vi "Boiler_Startup_Control.vi"() -> ()   [LabVIEW 2023]
doc: "This is the Main Vi that performs the boiler startup operation."
uses:
  Controls/Boiler_Status_Indicators.ctl
  Controls/Queue_Operation_Select.ctl
  Controls/Timer_Operation_Select.ctl
  Controls/Boiler_Data.ctl
  Controls/State_and_Data.ctl
  Controls/Notifier_Operation_Select.ctl
  <vilib>/Utility/file.llb/Write Delimited Spreadsheet (string).vi
panel:
  out "Boiler_Status_Indicators":T1 caption="Boiler Status Indicators"
  in  "Stop":bool
  in  "Forced_Draft_Fan":bool caption="Forced Draft Fan"
  in  "Run_Interlock":bool caption="Run Interlock"
  in  "Flame_Sensor_Value":dbl(slide) caption="Flame Sensor Value [%]" scale=0.0..100.0
  in  "Fuel_Control_Valve":dbl(knob) caption="Fuel  Control Valve Position [% Open]" scale=0.0..100.0 scale format="%.1f"
  in  "Shutdown":bool
  in  "Pilot":bool
  in  "Start_Sequence":bool caption="Start Sequence"
  in  "Boiler_Reset":bool caption="Boiler Reset"
  out "Error_Out":errorcluster
  in  "Error_In":errorcluster
  # "Boiler Controls"
  # "Boiler Simulation Controls"
  # "Closed"
  # "On"
  # "Open"
  # "Off"
  # "Boiler Start-Up steps\nStep1 : Close the interlock and hit the reset button.\nStep2 : Press the start sequence to initiate the pre-purge. \nStep3 : After the pre-purge, press the pilot button to turn on the natural gas and pilot.\nStep4 : Adjust the flame sensor to prepare the boiler.\nStep5 : Turn on the forced draft fan, then add fuel to the boiler by adjusting the fuel control valve.\nStep6 :The boiler is now started up"
  # "Seconds"
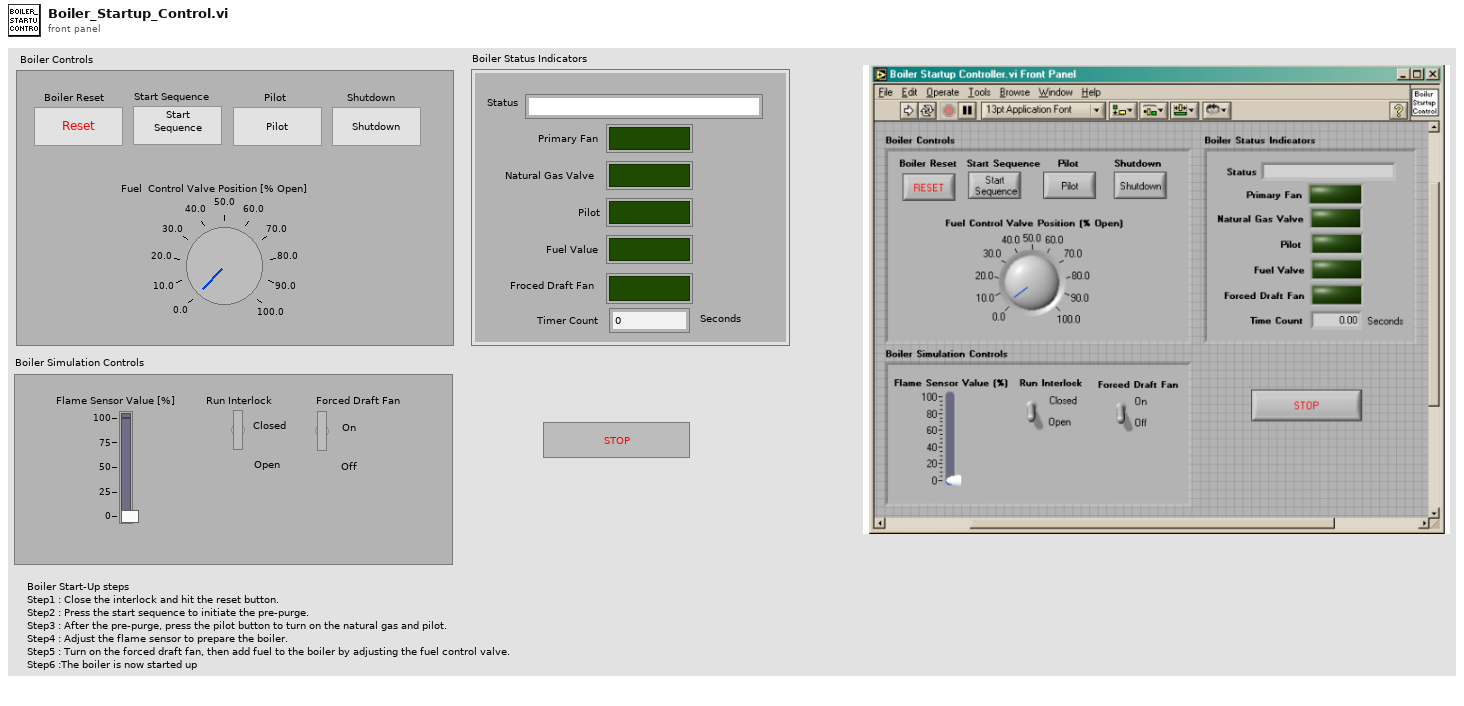
[diagram p1: front panel]
types:
  T1 = typedef "Boiler_Status_Indicators.ctl" = cluster{"Status":string, "Primary_Fan":bool, "Natural_Gas_Valve":bool, "Pilot":bool, "Fuel_Value":bool, "Froced_Draft_Fan":bool, "Timer_Count":dbl}
  T2 = typedef "Notifier_Operation_Select.ctl" = enum16{"Obtain_Notifier", "Send_Notification", "Get_Notification_Status", "Release_Notifier"}
  T3 = typedef "Queue_Operation_Select.ctl" = enum16{"Obtain_Queue", "Enqueue", "Enqueue_N", "Enqueue_at_First", "Dequeue", "Flush_Queue", "Release_Queue"}
  T4 = typedef "State_and_Data.ctl" = cluster{"State":string, "Event_Data":variant}
  T5 = typedef "Boiler_Data.ctl" = cluster{"Boiler_Status_Indicators":T1, "Start?":bool, "Pilot_On?":bool, "Blink_It?":bool, "Log_Timer_Time":bool, "ReInitialize":refnum<vi>[], "After_TimeOut_Call?":string, "Time_String":string, "Event_String":string, "Event_Data_String":string}
  T6 = typedef "Timer_Operation_Select.ctl" = enum16{"Start_Timer", "Pause_Timer", "Time_Out?", "Stop_Timer"}
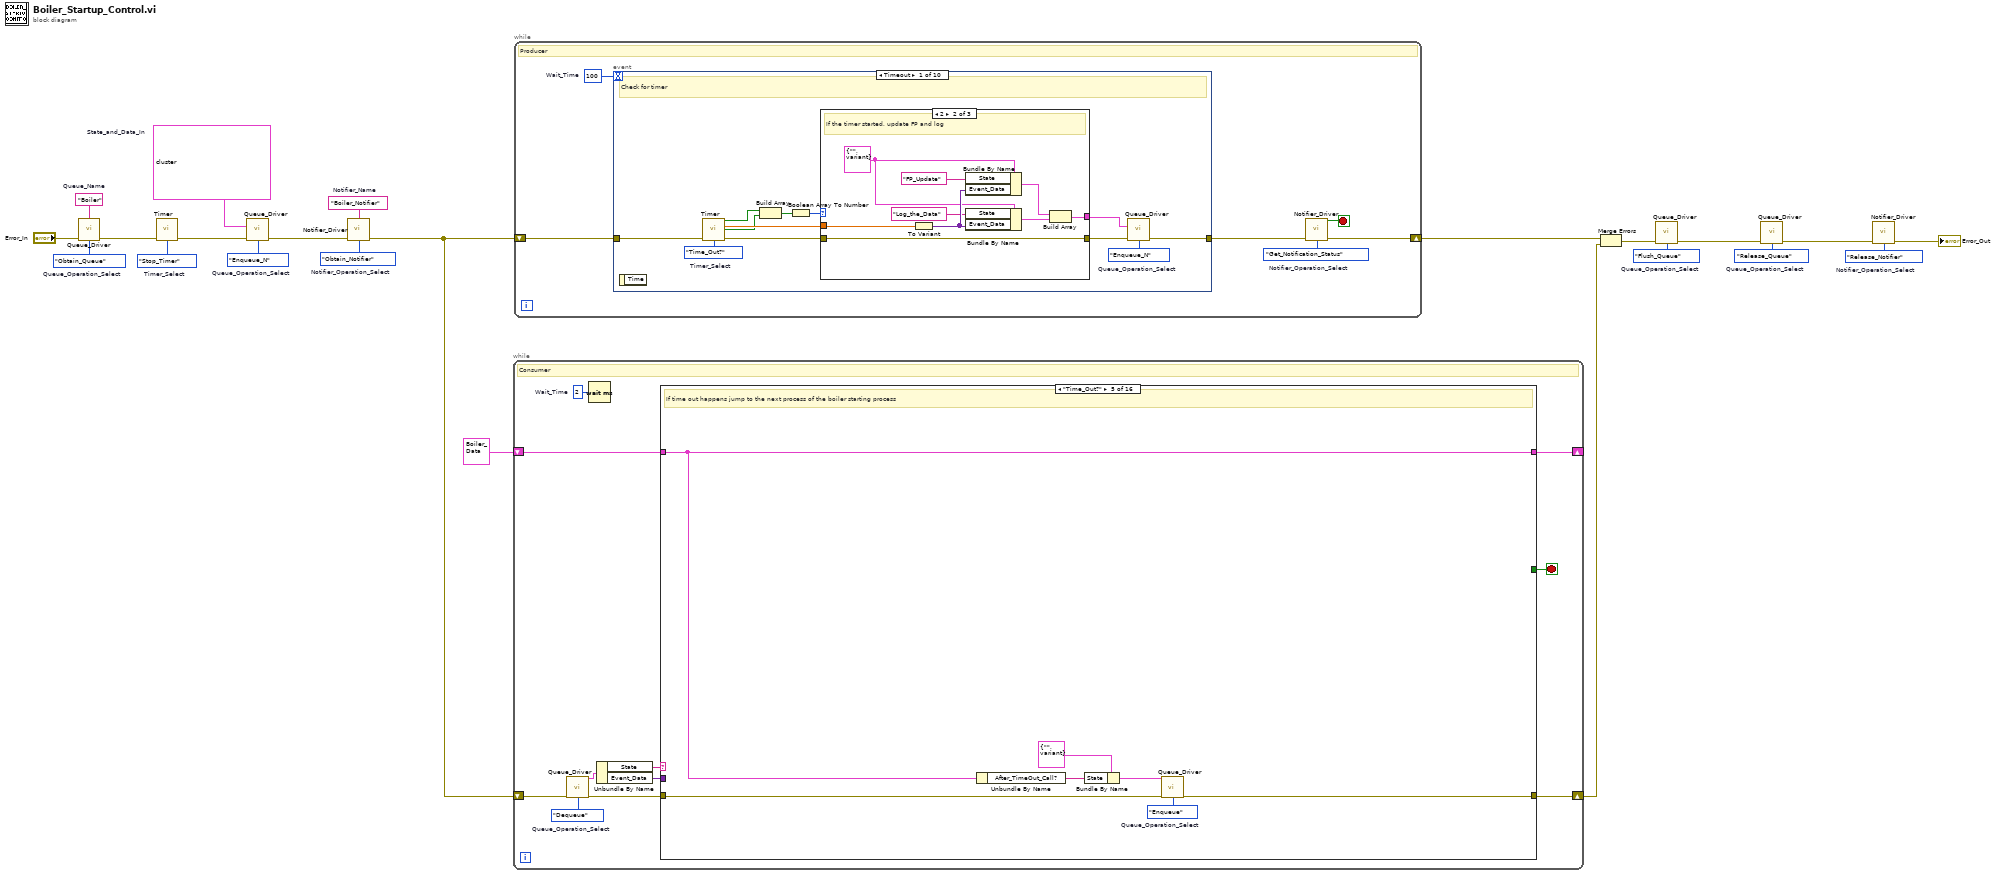
[diagram p0: block diagram]
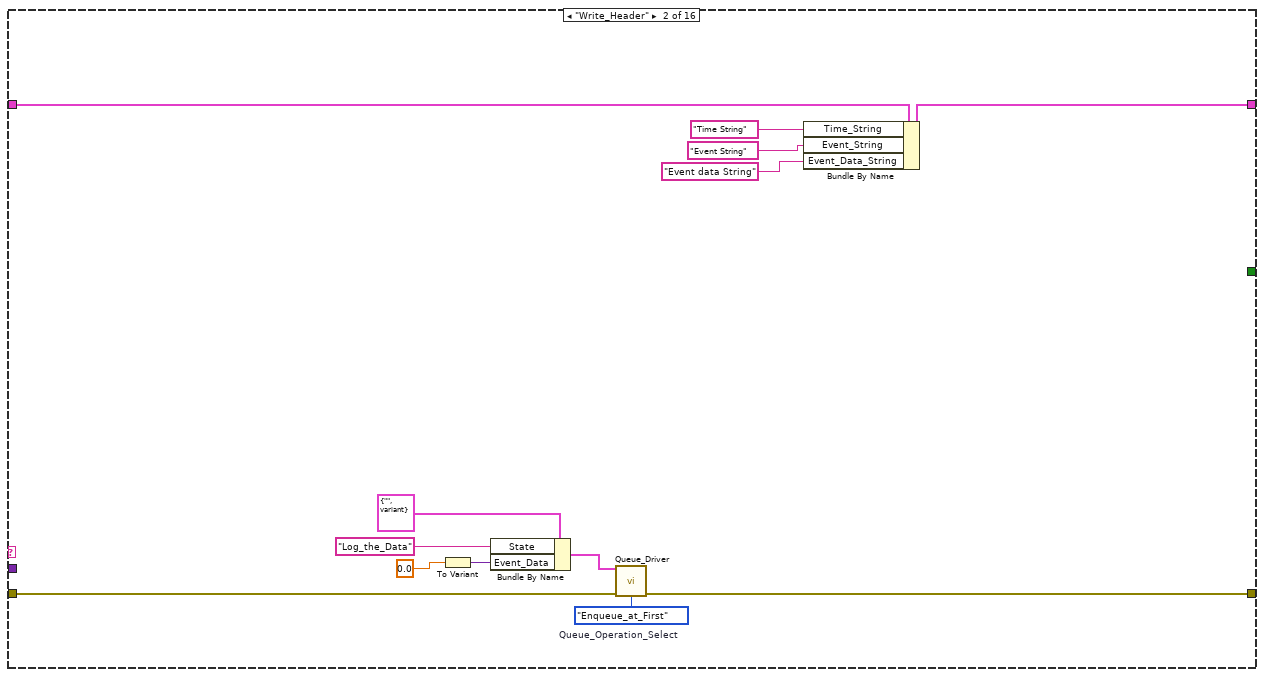
[diagram p3: hidden frame]
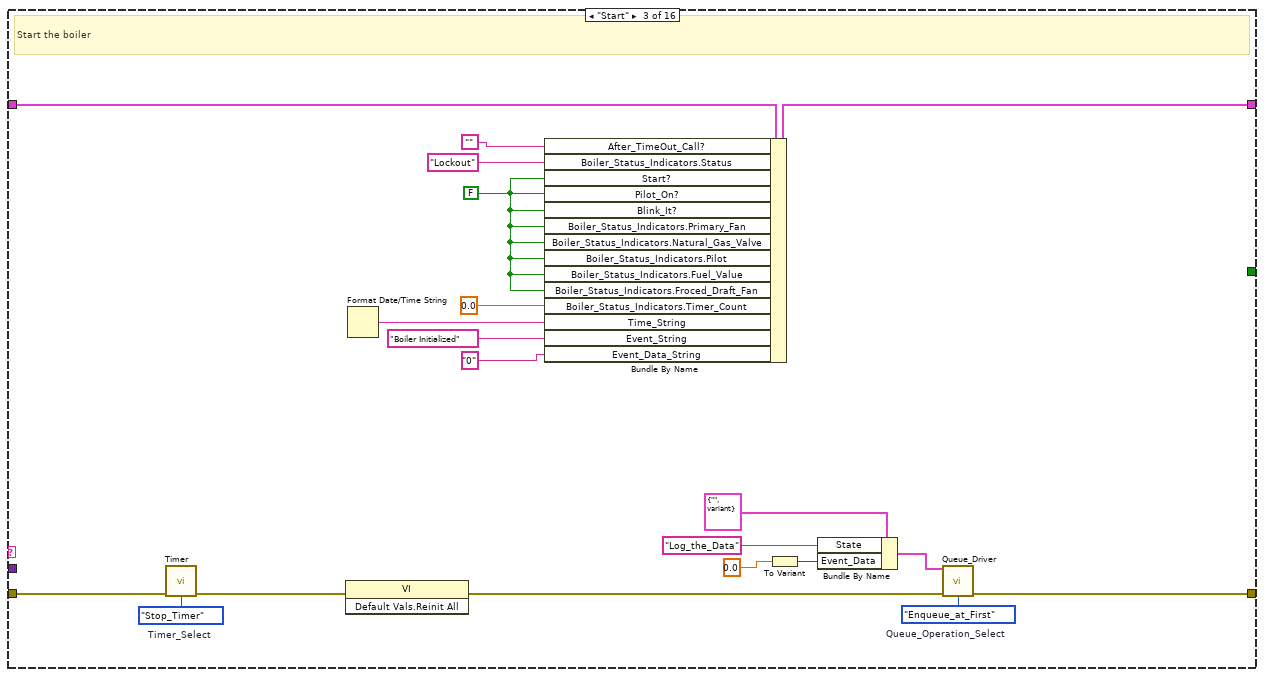
[diagram p4: hidden frame]
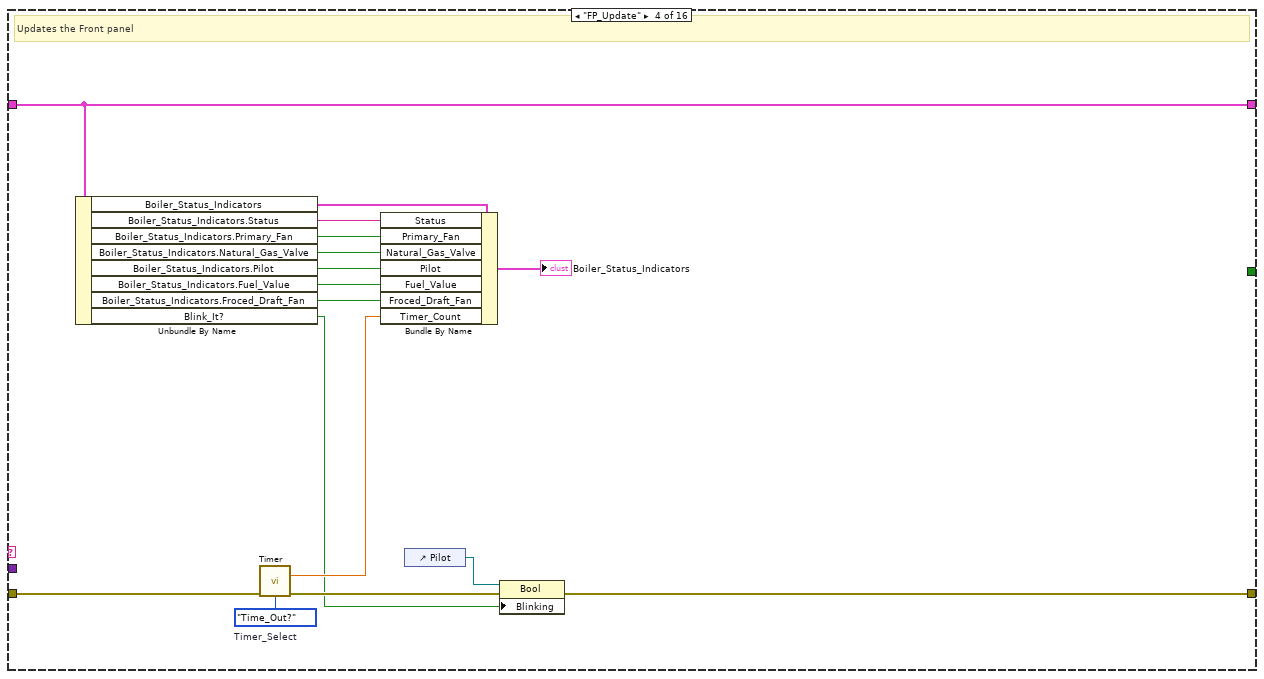
[diagram p5: hidden frame]
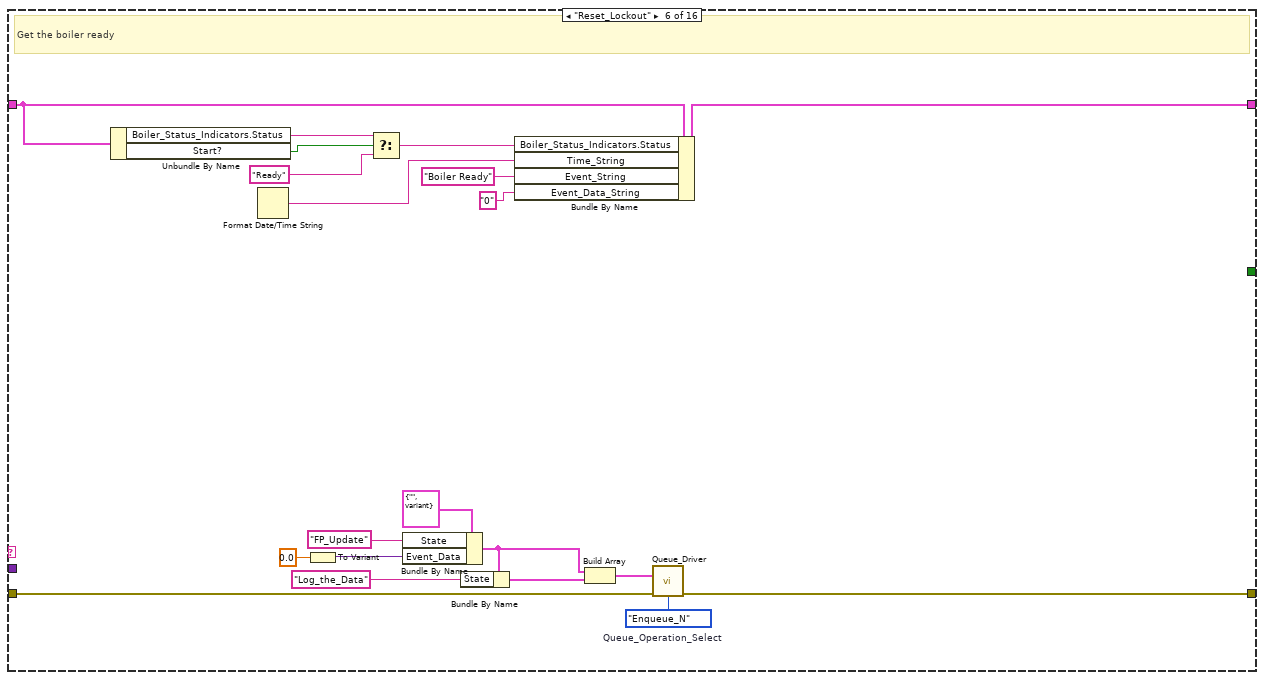
[diagram p6: hidden frame]
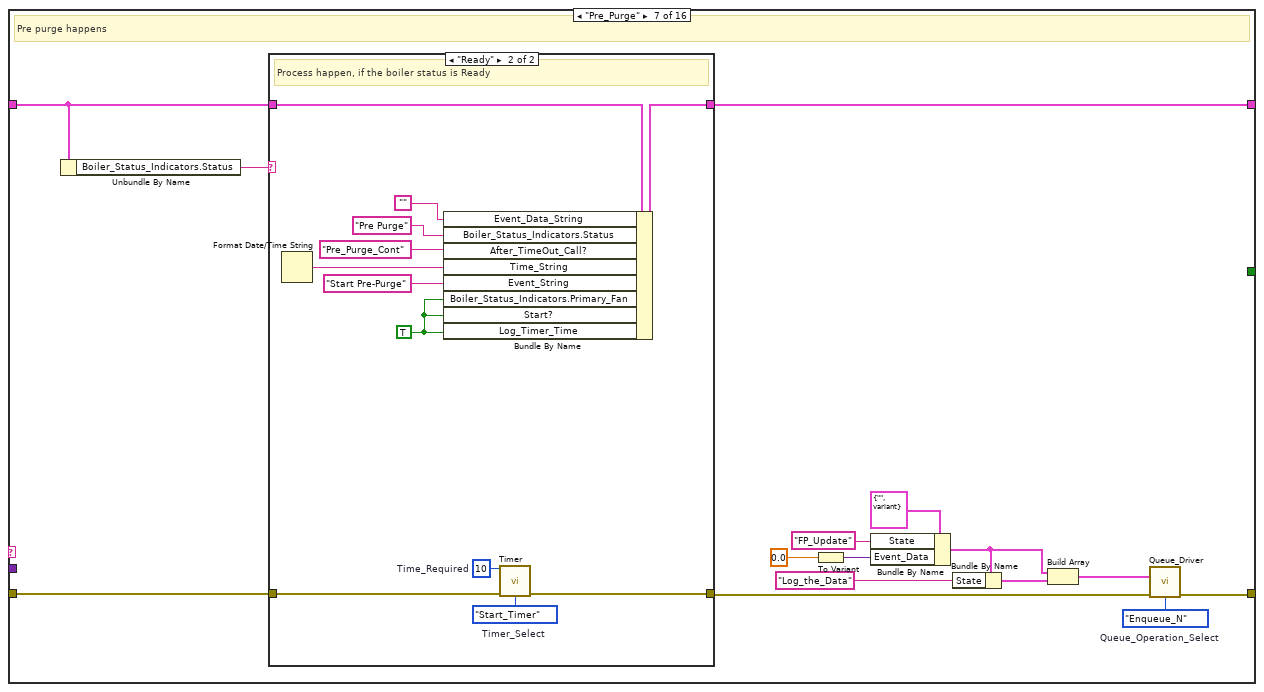
[diagram p7: hidden frame]
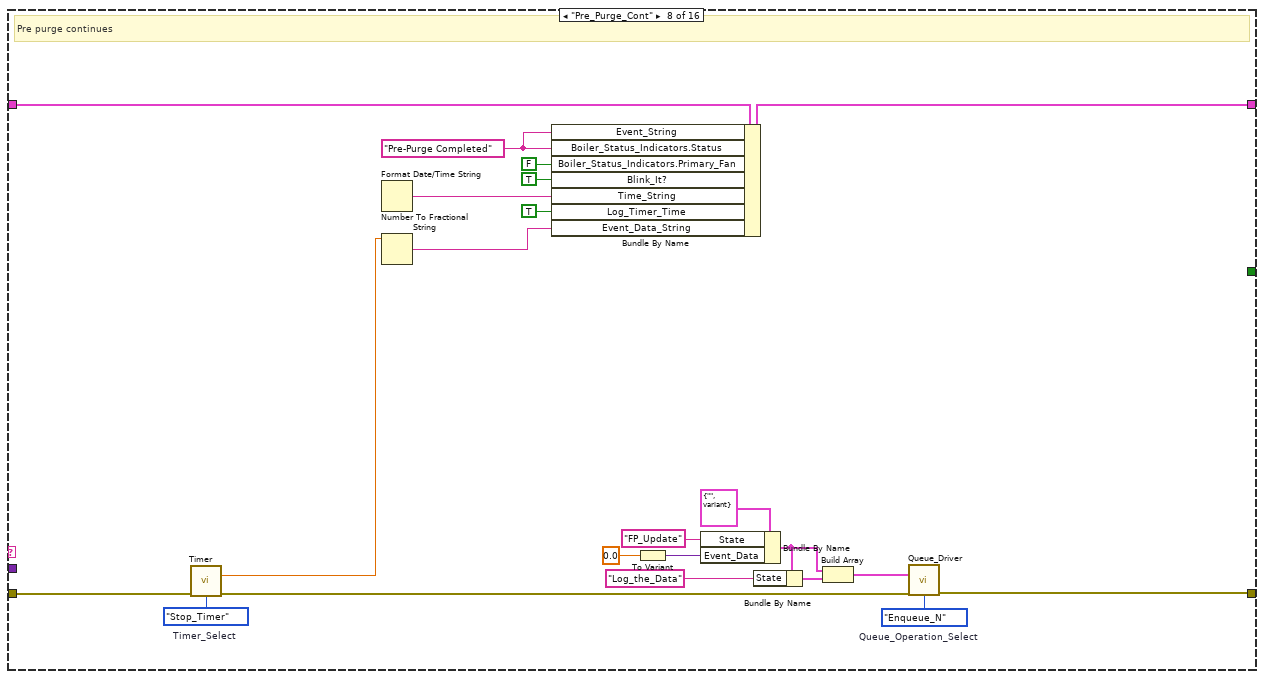
[diagram p9: hidden frame]
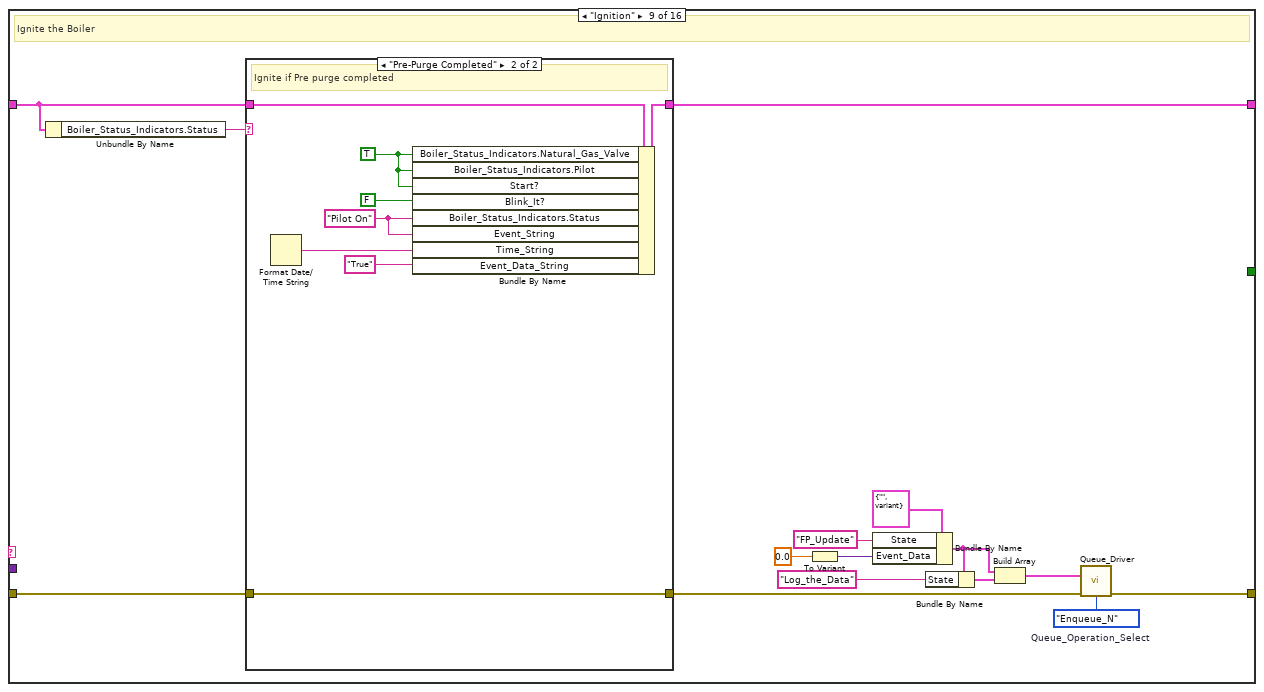
[diagram p10: hidden frame]
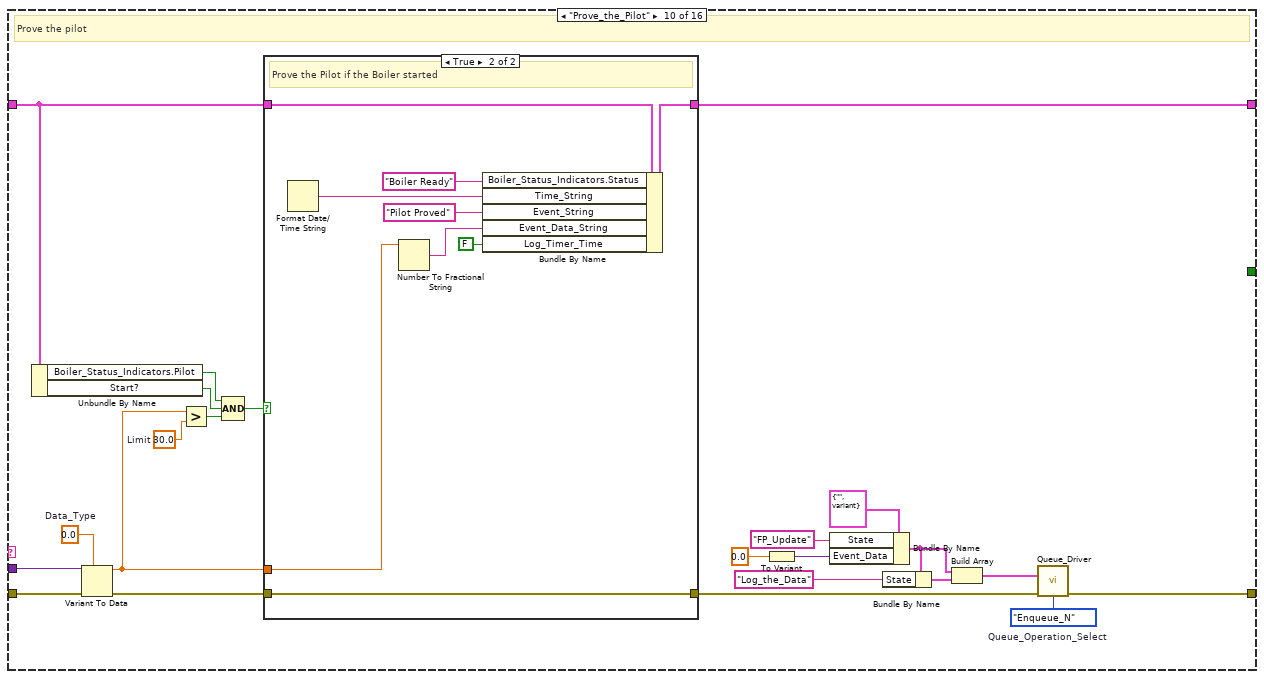
[diagram p12: hidden frame]
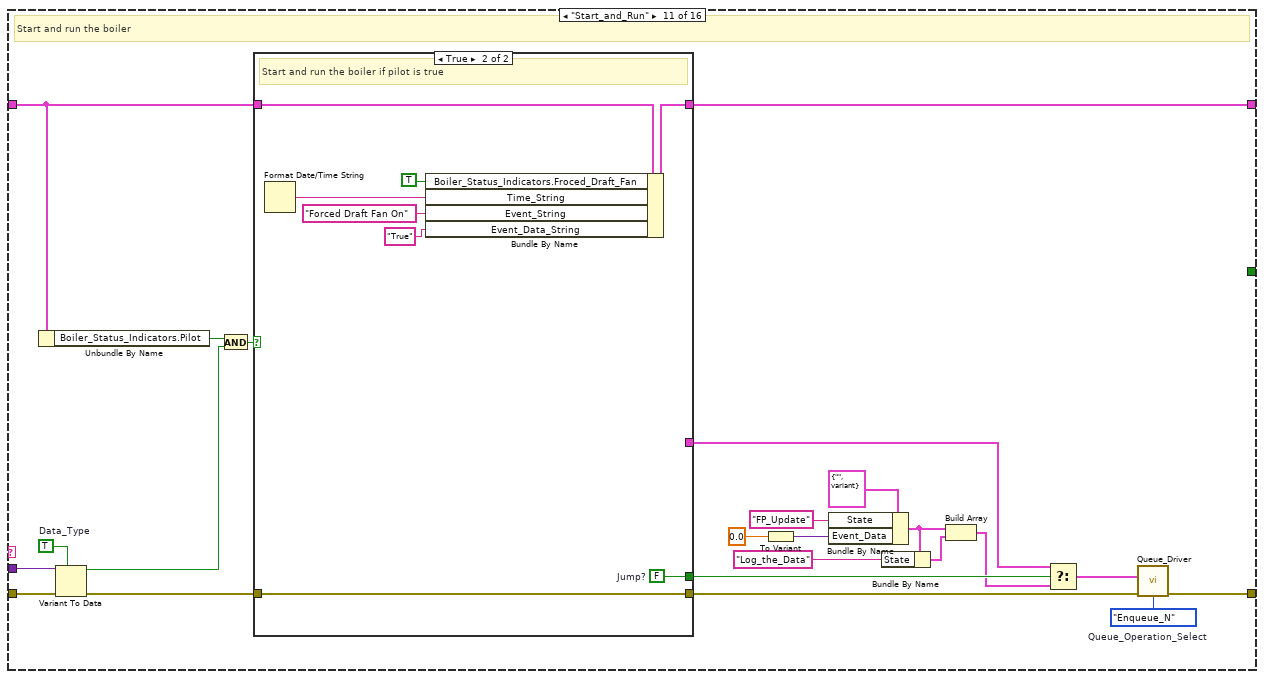
[diagram p14: hidden frame]
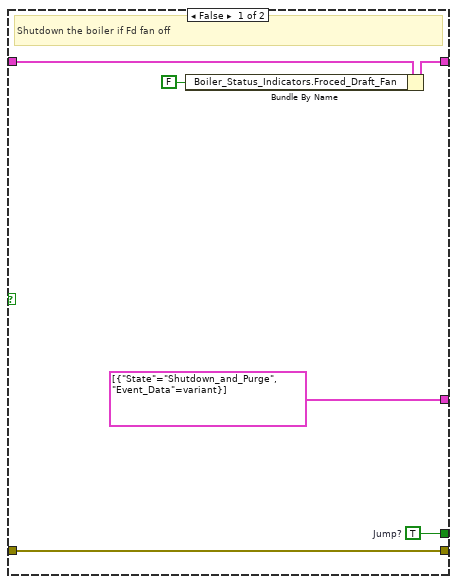
[diagram p15: hidden frame]
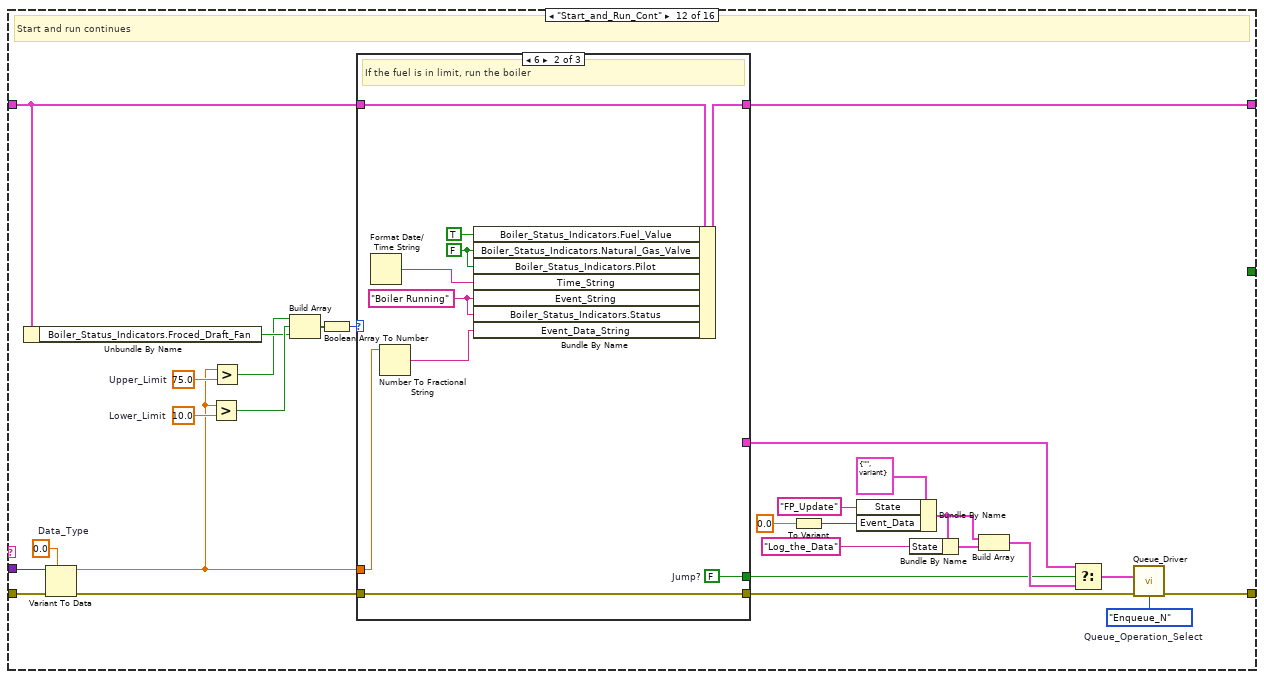
[diagram p16: hidden frame]
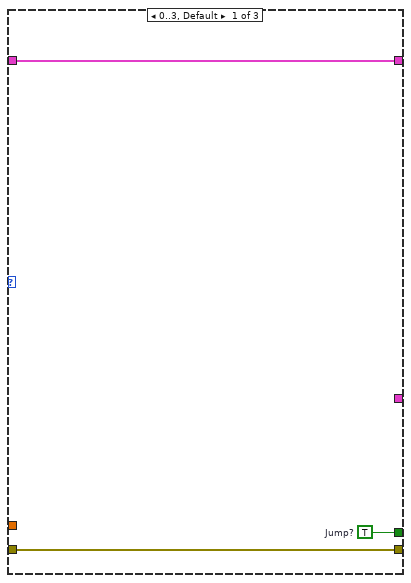
[diagram p17: hidden frame]
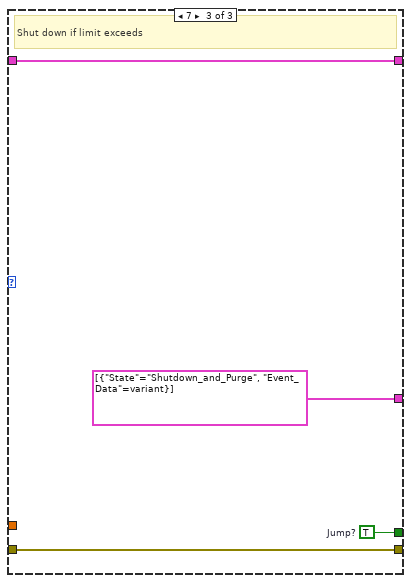
[diagram p18: hidden frame]
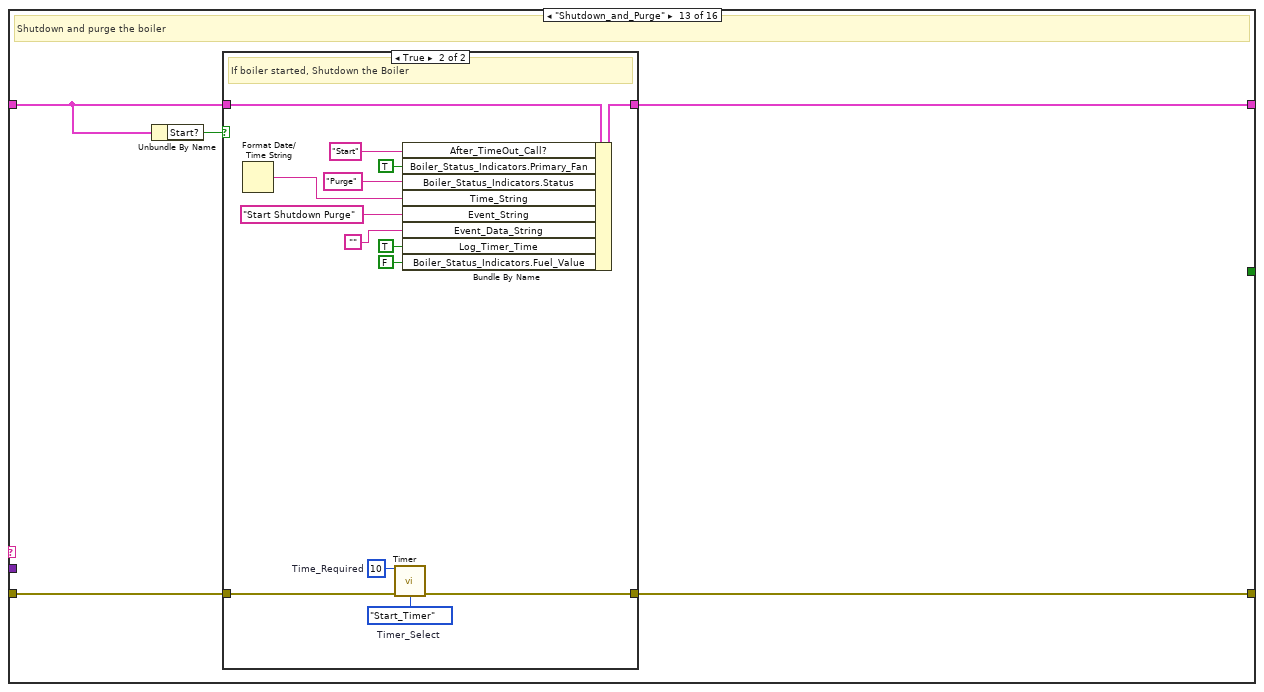
[diagram p19: hidden frame]
diagram:
  w5 = Notifier_Operation_Select."Release_Notifier"  # Notifier_Operation_Select
  w6 = Queue_Operation_Select."Release_Queue"  # Queue_Operation_Select
  w8 = Queue_Operation_Select."Flush_Queue"  # Queue_Operation_Select
  w10 = "Boiler_Notifier"  # Notifier_Name
  w11 = Notifier_Operation_Select."Obtain_Notifier"  # Notifier_Operation_Select
  w13 = T4[] [{"State"="Write_Header", "Event_Data"=variant}, {"State"="Start", "Event_Data"=variant}, {"State"="FP_Update", "Event_Data"=variant}]  # State_and_Data_In
  w14 = Queue_Operation_Select."Enqueue_N"  # Queue_Operation_Select
  w18 = Timer_Operation_Select."Stop_Timer"  # Timer_Select
  w19 = "Boiler"  # Queue_Name
  w20 = Queue_Operation_Select."Obtain_Queue"  # Queue_Operation_Select
  n1 = call "Queue_Driver.vi"("Queue_Name"=w19, "Error_In"="Error_In", "Queue_Operation_Select"=w20) -> ("Error_Out"=w21:errorcluster)  [unwired: 11 in, 1 out]
  n2 = call "Timer.vi"("Error_In"=w21, "Timer_Select"=w18) -> ("Error_Out"=w17:errorcluster)  [unwired: 10 in, 3 out]
  n3 = call "Queue_Driver.vi"("State_and_Data_In_N"=w13, "Error_In"=w17, "Queue_Operation_Select"=w14) -> ("Error_Out"=w15:errorcluster)  [unwired: 11 in, 1 out]
  n4 = call "Notifier_Driver.vi"("Notifier_Name"=w10, "Error_In"=w15, "Notifier_Operation_Select"=w11) -> ("Error_Out"=w12:errorcluster)  [unwired: 11 in, 1 out]
  n5 = while {
    shift-right: [w28] -> _
    shift-left: T5 {"Boiler_Status_Indicators"={"Status"="", "Primary_Fan"=FALSE, "Natural_Gas_Valve"=FALSE, "Pilot"=FALSE, "Fuel_Value"=FALSE, "Froced_Draft_Fan"=FALSE, "Timer_Count"=0.0}, "Start?"=TRUE, "Pilot_On?"=TRUE, "Blink_It?"=TRUE, "Log_Timer_Time"=FALSE, "ReInitialize"=[], "After_TimeOut_Call?"="", "Time_String"="", "Event_String"="", "Event_Data_String"=""} -> [w27]
    shift-right: [w23] -> w4
    shift-left: w12 -> [w33]
    stop <- w25 stop-if-true
    w24 = u32 2  # Wait_Time
    w31 = Queue_Operation_Select."Dequeue"  # Queue_Operation_Select
    # "Consumer"
    n6 = call "Queue_Driver.vi"("Error_In"=w33, "Queue_Operation_Select"=w31) -> ("State_and_Data_Out"=w30:T4, "Error_Out"=w32:errorcluster)  [unwired: 12 in]
    n7 = Wait (ms)(milliseconds to wait=w24) -> ()  [unwired: 1 out]
    n8 = Unbundle By Name(w30) -> ("State"=w29:string, "Event_Data"=w26:variant)
    n9 = case shown="\"Time_Out?\"" w29 {
      tunnel: w32 -> [w35 w48 w61 w84 w88 w95 w125 w159 w176 w210 w244 w284 w308 w343 w355 w364]
      tunnel: [w35 w42 w49 w69 w87 w94 w114 w141 w163 w189 w226 w262 w306 w347 w353 w359] -> w23
      tunnel: [w34 w46 w68 w83 w90 w111 w126 w162 w177 w201 w243 w286 w307 w344 w354 w375] -> w28
      tunnel: w27 -> [w34 w47 w67 w83 w90 w109 w124 w160 w175 w202 w242 w285 w305 w344 w354 w375]
      tunnel: w26 -> [_ _ _ _ _ _ _ _ _ w209 w239 w282 _ w342 _ _]
      tunnel: [_ _ _ _ _ _ _ _ _ _ _ _ _ _ w348 _] -> w25
      frame Default {
        # "Default"
      }
      frame "Write_Header" {
        w41 = Queue_Operation_Select."Enqueue_at_First"  # Queue_Operation_Select
        n10 = To Variant(anything=0.0) -> (Variant=w36:variant)
        n11 = Bundle By Name(cluster=T4 {"State"="", "Event_Data"=variant} ("State_and_Data_In"), "State"="Log_the_Data", "Event_Data"=w36) -> (w39:T4)
        n12 = call "Queue_Driver.vi"("State_and_Data_In"=w39, "Error_In"=w48, "Queue_Operation_Select"=w41) -> ("Error_Out"=w42:errorcluster)  [unwired: 11 in, 1 out]
        n13 = Bundle By Name(cluster=w47, "Time_String"="Time String", "Event_String"="Event String", "Event_Data_String"="Event data String") -> (w46:T5)
      }
      frame "Start" {
        w56 = Queue_Operation_Select."Enqueue_at_First"  # Queue_Operation_Select
        w58 = Timer_Operation_Select."Stop_Timer"  # Timer_Select
        w62 = FALSE ("Boiler_Status_Indicators.Primary_Fan")
        # "Start the boiler"
        n14 = call "Timer.vi"("Error_In"=w61, "Timer_Select"=w58) -> ("Error_Out"=w59:errorcluster)  [unwired: 10 in, 3 out]
        n15 = invoke on="Invoke Node" class="VI" method="Default Vals.Reinit All"(error in=w59) -> (error out=w50:errorcluster)  [unwired: 2 in, 2 out]
        n16 = Format Date/Time String() -> (date/time string=w57:string)  [unwired: 3 in]
        n17 = Bundle By Name(cluster=w67, "After_TimeOut_Call?"="" ("Empty String Constant"), "Boiler_Status_Indicators.Status"="Lockout", "Start?"=w62, "Pilot_On?"=w62, "Blink_It?"=w62, "Boiler_Status_Indicators.Primary_Fan"=w62, "Boiler_Status_Indicators.Natural_Gas_Valve"=w62, "Boiler_Status_Indicators.Pilot"=w62, "Boiler_Status_Indicators.Fuel_Value"=w62, "Boiler_Status_Indicators.Froced_Draft_Fan"=w62, "Boiler_Status_Indicators.Timer_Count"=0.0, "Time_String"=w57, "Event_String"="Boiler Initialized", "Event_Data_String"="0") -> (w68:T5)
        n18 = To Variant(anything=0.0) -> (Variant=w51:variant)
        n19 = Bundle By Name(cluster=T4 {"State"="", "Event_Data"=variant} ("State_and_Data_In"), "State"="Log_the_Data", "Event_Data"=w51) -> (w54:T4)
        n20 = call "Queue_Driver.vi"("State_and_Data_In"=w54, "Error_In"=w50, "Queue_Operation_Select"=w56) -> ("Error_Out"=w49:errorcluster)  [unwired: 11 in, 1 out]
      }
      frame "FP_Update" {
        w74 = Timer_Operation_Select."Time_Out?"  # Timer_Select
        # "Updates the Front panel"
        n21 = Unbundle By Name(w83) -> ("Boiler_Status_Indicators"=w82:T1, "Boiler_Status_Indicators.Status"=w81:string, "Boiler_Status_Indicators.Primary_Fan"=w80:bool, "Boiler_Status_Indicators.Natural_Gas_Valve"=w79:bool, "Boiler_Status_Indicators.Pilot"=w78:bool, "Boiler_Status_Indicators.Fuel_Value"=w77:bool, "Boiler_Status_Indicators.Froced_Draft_Fan"=w76:bool, "Blink_It?"=w71:bool)
        n22 = call "Timer.vi"("Error_In"=w84, "Timer_Select"=w74) -> ("Time"=w72:dbl, "Error_Out"=w75:errorcluster)  [unwired: 10 in, 2 out]
        n23 = Bundle By Name(cluster=w82, "Status"=w81, "Primary_Fan"=w80, "Natural_Gas_Valve"=w79, "Pilot"=w78, "Fuel_Value"=w77, "Froced_Draft_Fan"=w76, "Timer_Count"=w72) -> (→"Boiler_Status_Indicators":T1)
        n24 = control-ref of="Pilot"() -> (w70:refnum<vi>)
        n25 = property on="Property Node" class="Bool"(reference=w70, error in=w75, "Blinking"=w71) -> (error out=w69:errorcluster)  [unwired: 1 out]
      }
      frame "Time_Out?" {
        w86 = Queue_Operation_Select."Enqueue"  # Queue_Operation_Select
        # "If time out happens jump to the next process of the boiler starting process"
        n26 = Unbundle By Name(w90) -> ("After_TimeOut_Call?"=w91:string)
        n27 = Bundle By Name(cluster=T4 {"State"="", "Event_Data"=variant} ("State_and_Data_In"), "State"=w91) -> (w85:T4)
        n28 = call "Queue_Driver.vi"("State_and_Data_In"=w85, "Error_In"=w88, "Queue_Operation_Select"=w86) -> ("Error_Out"=w87:errorcluster)  [unwired: 11 in, 1 out]
      }
      frame "Reset_Lockout" {
        w103 = Queue_Operation_Select."Enqueue_N"  # Queue_Operation_Select
        # "Get the boiler ready"
        n29 = Unbundle By Name(w109) -> ("Boiler_Status_Indicators.Status"=w106:string, "Start?"=w107:bool)
        n30 = Format Date/Time String() -> (date/time string=w104:string)  [unwired: 3 in]
        n31 = To Variant(anything=0.0) -> (Variant=w98:variant)
        n32 = Select(t=w106, s=w107, f="Ready") -> (s? t:f=w108:string)
        n33 = Bundle By Name(cluster=T4 {"State"="", "Event_Data"=variant} ("State_and_Data_In"), "State"="FP_Update", "Event_Data"=w98) -> (w96:T4)
        n34 = Bundle By Name(cluster=w96, "State"="Log_the_Data") -> (w97:T4)
        n35 = Bundle By Name(cluster=w109, "Boiler_Status_Indicators.Status"=w108, "Time_String"=w104, "Event_String"="Boiler Ready", "Event_Data_String"="0") -> (w111:T5)
        n36 = Build Array(w96, w97) -> (w93:T4[])
        n37 = call "Queue_Driver.vi"("State_and_Data_In_N"=w93, "Error_In"=w95, "Queue_Operation_Select"=w103) -> ("Error_Out"=w94:errorcluster)  [unwired: 11 in, 1 out]
      }
      frame "Pre_Purge" {
        w116 = Queue_Operation_Select."Enqueue_N"  # Queue_Operation_Select
        # "Pre purge happens"
        n38 = Unbundle By Name(w124) -> ("Boiler_Status_Indicators.Status"=w123:string)
        n39 = case shown="\"Ready\"" w123 {
          tunnel: w124 -> [w128 w140]
          tunnel: [w128 w139] -> w126
          tunnel: w125 -> [w127 w136]
          tunnel: [w127 w135] -> w115
          frame Default {
          }
          frame "Ready" {
            w131 = TRUE ("Log_Timer_Time")
            w137 = 10  # Time_Required
            w138 = Timer_Operation_Select."Start_Timer"  # Timer_Select
            # "Process happen, if the boiler status is Ready"
            n40 = Format Date/Time String() -> (date/time string=w129:string)  [unwired: 3 in]
            n41 = Bundle By Name(cluster=w140, "Event_Data_String"="" ("Empty String Constant"), "Boiler_Status_Indicators.Status"="Pre Purge", "After_TimeOut_Call?"="Pre_Purge_Cont", "Time_String"=w129, "Event_String"="Start Pre-Purge", "Boiler_Status_Indicators.Primary_Fan"=w131, "Start?"=w131, "Log_Timer_Time"=w131) -> (w139:T5)
            n42 = call "Timer.vi"("Time_Required"=w137, "Error_In"=w136, "Timer_Select"=w138) -> ("Error_Out"=w135:errorcluster)  [unwired: 9 in, 3 out]
          }
        }
        n43 = To Variant(anything=0.0) -> (Variant=w120:variant)
        n44 = Bundle By Name(cluster=T4 {"State"="", "Event_Data"=variant} ("State_and_Data_In"), "State"="FP_Update", "Event_Data"=w120) -> (w122:T4)
        n45 = Bundle By Name(cluster=w122, "State"="Log_the_Data") -> (w121:T4)
        n46 = Build Array(w122, w121) -> (w113:T4[])
        n47 = call "Queue_Driver.vi"("State_and_Data_In_N"=w113, "Error_In"=w115, "Queue_Operation_Select"=w116) -> ("Error_Out"=w114:errorcluster)  [unwired: 11 in, 1 out]
      }
      frame "Pre_Purge_Cont" {
        w147 = Queue_Operation_Select."Enqueue_N"  # Queue_Operation_Select
        w158 = Timer_Operation_Select."Stop_Timer"  # Timer_Select
        w156 = "Pre-Purge Completed" ("Boiler_Status_Indicators.Status")
        # "Pre purge continues"
        n48 = call "Timer.vi"("Error_In"=w159, "Timer_Select"=w158) -> ("Time"=w143:dbl, "Error_Out"=w142:errorcluster)  [unwired: 10 in, 2 out]
        n49 = Format Date/Time String() -> (date/time string=w154:string)  [unwired: 3 in]
        n50 = Number To Fractional String(number=w143) -> (F-format string=w144:string)  [unwired: 3 in]
        n51 = Bundle By Name(cluster=w160, "Event_String"=w156, "Boiler_Status_Indicators.Status"=w156, "Boiler_Status_Indicators.Primary_Fan"=FALSE, "Blink_It?"=TRUE, "Time_String"=w154, "Log_Timer_Time"=TRUE, "Event_Data_String"=w144) -> (w162:T5)
        n52 = To Variant(anything=0.0) -> (Variant=w151:variant)
        n53 = Bundle By Name(cluster=T4 {"State"="", "Event_Data"=variant} ("State_and_Data_In"), "State"="FP_Update", "Event_Data"=w151) -> (w153:T4)
        n54 = Bundle By Name(cluster=w153, "State"="Log_the_Data") -> (w152:T4)
        n55 = Build Array(w153, w152) -> (w146:T4[])
        n56 = call "Queue_Driver.vi"("State_and_Data_In_N"=w146, "Error_In"=w142, "Queue_Operation_Select"=w147) -> ("Error_Out"=w141:errorcluster)  [unwired: 11 in, 1 out]
      }
      frame "Ignition" {
        w167 = Queue_Operation_Select."Enqueue_N"  # Queue_Operation_Select
        # "Ignite the Boiler"
        n57 = Unbundle By Name(w175) -> ("Boiler_Status_Indicators.Status"=w174:string)
        n58 = case shown="\"Pre-Purge Completed\"" w174 {
          tunnel: w175 -> [w178 w187]
          tunnel: [w178 w186] -> w177
          tunnel: [w179 w185] -> w164
          tunnel: w176 -> [w179 w185]
          frame Default {
          }
          frame "Pre-Purge Completed" {
            w183 = "Pilot On" ("Boiler_Status_Indicators.Status")
            w184 = TRUE ("Boiler_Status_Indicators.Natural_Gas_Valve")
            # "Ignite if Pre purge completed"
            n59 = Format Date/Time String() -> (date/time string=w180:string)  [unwired: 3 in]
            n60 = Bundle By Name(cluster=w187, "Boiler_Status_Indicators.Natural_Gas_Valve"=w184, "Boiler_Status_Indicators.Pilot"=w184, "Start?"=w184, "Blink_It?"=FALSE, "Boiler_Status_Indicators.Status"=w183, "Event_String"=w183, "Time_String"=w180, "Event_Data_String"="True") -> (w186:T5)
          }
        }
        n61 = To Variant(anything=0.0) -> (Variant=w171:variant)
        n62 = Bundle By Name(cluster=T4 {"State"="", "Event_Data"=variant} ("State_and_Data_In"), "State"="FP_Update", "Event_Data"=w171) -> (w173:T4)
        n63 = Bundle By Name(cluster=w173, "State"="Log_the_Data") -> (w172:T4)
        n64 = Build Array(w173, w172) -> (w166:T4[])
        n65 = call "Queue_Driver.vi"("State_and_Data_In_N"=w166, "Error_In"=w164, "Queue_Operation_Select"=w167) -> ("Error_Out"=w163:errorcluster)  [unwired: 11 in, 1 out]
      }
      frame "Prove_the_Pilot" {
        w193 = Queue_Operation_Select."Enqueue_N"  # Queue_Operation_Select
        w206 = 30.0  # Limit
        w207 = 0.0  # Data_Type
        # "Prove the pilot"
        n66 = Unbundle By Name(w202) -> ("Boiler_Status_Indicators.Pilot"=w188:bool, "Start?"=w204:bool)
        n67 = Variant To Data(error in=w210, type=w207, Variant=w209) -> (data=w200:dbl, error out=w208:errorcluster)
        n68 = Greater?(x=w200, y=w206) -> (0:w205:bool)
        n69 = Compound Arithmetic op=AND(w188, w204, w205) -> (w203:bool)
        n70 = case shown="True" w203 {
          tunnel: [w212 w221] -> w190
          tunnel: w208 -> [w212 w221]
          tunnel: w202 -> [w211 w220]
          tunnel: [w211 w219] -> w201
          tunnel: w200 -> [_ w215]
          frame False {
          }
          frame True {
            # "Prove the Pilot if the Boiler started"
            n71 = Format Date/Time String() -> (date/time string=w213:string)  [unwired: 3 in]
            n72 = Number To Fractional String(number=w215) -> (F-format string=w216:string)  [unwired: 3 in]
            n73 = Bundle By Name(cluster=w220, "Boiler_Status_Indicators.Status"="Boiler Ready", "Time_String"=w213, "Event_String"="Pilot Proved", "Event_Data_String"=w216, "Log_Timer_Time"=FALSE) -> (w219:T5)
          }
        }
        n74 = To Variant(anything=0.0) -> (Variant=w197:variant)
        n75 = Bundle By Name(cluster=T4 {"State"="", "Event_Data"=variant} ("State_and_Data_In"), "State"="FP_Update", "Event_Data"=w197) -> (w199:T4)
        n76 = Bundle By Name(cluster=w199, "State"="Log_the_Data") -> (w198:T4)
        n77 = Build Array(w199, w198) -> (w192:T4[])
        n78 = call "Queue_Driver.vi"("State_and_Data_In_N"=w192, "Error_In"=w190, "Queue_Operation_Select"=w193) -> ("Error_Out"=w189:errorcluster)  [unwired: 11 in, 1 out]
      }
      frame "Start_and_Run" {
        w229 = Queue_Operation_Select."Enqueue_N"  # Queue_Operation_Select
        w238 = TRUE  # Data_Type
        # "Start and run the boiler"
        n79 = Unbundle By Name(w242) -> ("Boiler_Status_Indicators.Pilot"=w241:bool)
        n80 = Variant To Data(error in=w244, type=w238, Variant=w239) -> (data=w236:bool, error out=w240:errorcluster)
        n81 = And(x=w241, y=w236) -> (x .and. y?=w237:bool)
        n82 = case shown="True" w237 {
          tunnel: [w249 w258] -> w227
          tunnel: w240 -> [w249 w258]
          tunnel: [w246 w256] -> w243
          tunnel: w242 -> [w250 w257]
          tunnel: [T4[] [{"State"="Shutdown_and_Purge", "Event_Data"=variant}] _] -> w224
          tunnel: [w247 w252] -> w223
          frame False {
            w247 = TRUE  # Jump?
            # "Shutdown the boiler if Fd fan off"
            n83 = Bundle By Name(cluster=w250, "Boiler_Status_Indicators.Froced_Draft_Fan"=FALSE) -> (w246:T5)
          }
          frame True {
            w252 = FALSE  # Jump?
            # "Start and run the boiler if pilot is true"
            n84 = Format Date/Time String() -> (date/time string=w251:string)  [unwired: 3 in]
            n85 = Bundle By Name(cluster=w257, "Boiler_Status_Indicators.Froced_Draft_Fan"=TRUE, "Time_String"=w251, "Event_String"="Forced Draft Fan On", "Event_Data_String"="True") -> (w256:T5)
          }
        }
        n86 = To Variant(anything=0.0) -> (Variant=w233:variant)
        n87 = Bundle By Name(cluster=T4 {"State"="", "Event_Data"=variant} ("State_and_Data_In"), "State"="FP_Update", "Event_Data"=w233) -> (w235:T4)
        n88 = Bundle By Name(cluster=w235, "State"="Log_the_Data") -> (w234:T4)
        n89 = Build Array(w235, w234) -> (w222:T4[])
        n90 = Select(t=w224, s=w223, f=w222) -> (s? t:f=w225:T4[])
        n91 = call "Queue_Driver.vi"("State_and_Data_In_N"=w225, "Error_In"=w227, "Queue_Operation_Select"=w229) -> ("Error_Out"=w226:errorcluster)  [unwired: 11 in, 1 out]
      }
      frame "Start_and_Run_Cont" {
        w266 = Queue_Operation_Select."Enqueue_N"  # Queue_Operation_Select
        w278 = 10.0  # Lower_Limit
        w276 = 75.0  # Upper_Limit
        w281 = 0.0  # Data_Type
        # "Start and run continues"
        n92 = Unbundle By Name(w285) -> ("Boiler_Status_Indicators.Froced_Draft_Fan"=w274:bool)
        n93 = Variant To Data(error in=w284, type=w281, Variant=w282) -> (data=w275:dbl, error out=w283:errorcluster)
        n94 = Greater?(x=w275, y=w278) -> (0:w277:bool)
        n95 = Greater?(x=w275, y=w276) -> (0:w273:bool)
        n96 = Build Array(w273, w277, w274) -> (w280:bool[])
        n97 = Boolean Array To Number(Boolean array=w280) -> (number=w279:u32)
        n98 = case shown="6" w279 {
          tunnel: w285 -> [w288 w299 w303]
          tunnel: [w288 w298 w303] -> w286
          tunnel: [w289 w297 w302] -> w263
          tunnel: w283 -> [w289 w297 w302]
          tunnel: [_ _ T4[] [{"State"="Shutdown_and_Purge", "Event_Data"=variant}]] -> w259
          tunnel: w275 -> [_ w293 _]
          tunnel: [w287 w292 w300] -> w260
          frame 0..3, Default {
            w287 = TRUE  # Jump?
          }
          frame 6 {
            w292 = FALSE  # Jump?
            w290 = "Boiler Running" ("Event_String")
            w295 = FALSE ("Boiler_Status_Indicators.Natural_Gas_Valve")
            # "If the fuel is in limit, run the boiler"
            n99 = Format Date/Time String() -> (date/time string=w291:string)  [unwired: 3 in]
            n100 = Number To Fractional String(number=w293) -> (F-format string=w294:string)  [unwired: 3 in]
            n101 = Bundle By Name(cluster=w299, "Boiler_Status_Indicators.Fuel_Value"=TRUE, "Boiler_Status_Indicators.Natural_Gas_Valve"=w295, "Boiler_Status_Indicators.Pilot"=w295, "Time_String"=w291, "Event_String"=w290, "Boiler_Status_Indicators.Status"=w290, "Event_Data_String"=w294) -> (w298:T5)
          }
          frame 7 {
            w300 = TRUE  # Jump?
            # "Shut down if limit exceeds"
          }
        }
        n102 = To Variant(anything=0.0) -> (Variant=w270:variant)
        n103 = Bundle By Name(cluster=T4 {"State"="", "Event_Data"=variant} ("State_and_Data_In"), "State"="FP_Update", "Event_Data"=w270) -> (w272:T4)
        n104 = Bundle By Name(cluster=w272, "State"="Log_the_Data") -> (w271:T4)
        n105 = Build Array(w272, w271) -> (w265:T4[])
        n106 = Select(t=w259, s=w260, f=w265) -> (s? t:f=w261:T4[])
        n107 = call "Queue_Driver.vi"("State_and_Data_In_N"=w261, "Error_In"=w263, "Queue_Operation_Select"=w266) -> ("Error_Out"=w262:errorcluster)  [unwired: 11 in, 1 out]
      }
      frame "Shutdown_and_Purge" {
        # "Shutdown and purge the boiler"
        n108 = Unbundle By Name(w305) -> ("Start?"=w304:bool)
        n109 = case shown="True" w304 {
          tunnel: w308 -> [w309 w324]
          tunnel: w305 -> [w310 w323]
          tunnel: [w310 w322] -> w307
          tunnel: [w309 w321] -> w306
          frame False {
          }
          frame True {
            w319 = 10  # Time_Required
            w320 = Timer_Operation_Select."Start_Timer"  # Timer_Select
            # "If boiler started, Shutdown the Boiler"
            n110 = Format Date/Time String() -> (date/time string=w314:string)  [unwired: 3 in]
            n111 = call "Timer.vi"("Time_Required"=w319, "Error_In"=w324, "Timer_Select"=w320) -> ("Error_Out"=w321:errorcluster)  [unwired: 9 in, 3 out]
            n112 = Bundle By Name(cluster=w323, "After_TimeOut_Call?"="Start", "Boiler_Status_Indicators.Primary_Fan"=TRUE, "Boiler_Status_Indicators.Status"="Purge", "Time_String"=w314, "Event_String"="Start Shutdown Purge", "Event_Data_String"="", "Log_Timer_Time"=TRUE, "Boiler_Status_Indicators.Fuel_Value"=FALSE) -> (w322:T5)
          }
        }
      }
      frame "Log_the_Data" {
        w341 = 0.0  # Data_Type
        w345 = path "Boiler Log.txt"  # File_Path
        w346 = ","  # Delimiter
        # "Log the boiler data"
        n113 = Unbundle By Name(w344) -> ("Time_String"=w340:string, "Event_String"=w339:string, "Event_Data_String"=w335:string, "Log_Timer_Time"=w333:bool)
        n114 = Variant To Data(error in=w343, type=w341, Variant=w342) -> (data=w338:dbl, error out=w326:errorcluster)
        n115 = Number To Fractional String(number=w338) -> (F-format string=w337:string)  [unwired: 3 in]
        n116 = Empty String/Path?(string/path=w335) -> (empty?=w334:bool)
        n117 = And(x=w334, y=w333) -> (x .and. y?=w332:bool)
        n118 = Select(t=w337, s=w332, f=w335) -> (s? t:f=w336:string)
        n119 = Build Array(w340, w339, w336) -> (w325:string[])
        n120 = call <vilib>:"Application Directory.vi"() -> ("Application Directory"=w327:path)
        n121 = Build Path(base path=w327, name or relative path=w345) -> (appended path=w330:path)
        n122 = call <vilib>:"Check if File or Folder Exists.vi"("error in (no error)"=w326, "path"=w330) -> ("error out"=w331:errorcluster, "file or folder exists?"=w328:bool, "dup path"=w329:path)  [unwired: 7 in]
        n123 = call-poly <vilib>:"Write Delimited Spreadsheet.vi"("file path (dialog if empty)"=w329, "1D data"=w325, "append to file? (new file:F)"=w328, "error in (no error)"=w331, "delimiter (\\t)"=w346) -> ("error out"=w347:errorcluster)  [unwired: 9 in, 1 out]
      }
      frame "Exit" {
        w351 = "No"  # Back
        w350 = "Yes"  # Stop_Execution
        w352 = Notifier_Operation_Select."Send_Notification"  # Notifier_Operation_Select
        # "Close the Application"
        n124 = disable-structure "Conditional Disable Structure" shown="RUN_TIME_ENGINE==True" {
          disable-tunnel: [w356 "Do you want to Exit" ("Message")] -> w349
          frame condition #0 (active) {
            w356 = "Do you want to stop the execution"  # Message
            # "Developer mode"
          }
          frame condition #1 {
            # "Run time engine mode"
          }
        }
        n125 = Two Button Dialog(message=w349, 1:w351, 2:w350) -> (T button?=w348:bool)
        n126 = call "Notifier_Driver.vi"("Notification"=w348, "Error_In"=w355, "Notifier_Operation_Select"=w352) -> ("Error_Out"=w353:errorcluster)  [unwired: 11 in, 1 out]
      }
      frame "Error" {
        w361 = Queue_Operation_Select."Enqueue_N"  # Queue_Operation_Select
        w369 = "%d%s%s"  # Format_String
        w370 = "Application Error"  # Initial_String
        w371 = "Stop"  # T_Button
        w372 = "Continue"  # F_Button
        w374 = T4[] [{"State"="Exit", "Event_Data"=variant}]  # State_and_Data_In
        # "Handles the error"
        n127 = call <vilib>:"Clear Errors.vi"("error in (no error)"=w364) -> ("error out"=w367:errorcluster)  [unwired: 5 in, 1 out]
        n128 = Unbundle By Name(w364) -> ("code"=w366:i32, "source"=w365:string)
        n129 = Format Into String(format string=w369, initial string=w370, error in=w367, w366, "\n" ("Line Feed Constant"), w365) -> (resulting string=w373:string, error out=w360:errorcluster)
        n130 = Two Button Dialog(message=w373, 1:w372, 2:w371) -> (T button?=w363:bool)
        n131 = Select(t=w374, s=w363, f=T4[] []) -> (s? t:f=w358:T4[])
        n132 = call "Queue_Driver.vi"("State_and_Data_In_N"=w358, "Error_In"=w360, "Queue_Operation_Select"=w361) -> ("Error_Out"=w359:errorcluster)  [unwired: 11 in, 1 out]
      }
    }
  }
  n133 = while {
    shift-right: [w376] -> w3
    shift-left: w12 -> [w381]
    stop <- w378 stop-if-true
    w379 = Notifier_Operation_Select."Get_Notification_Status"  # Notifier_Operation_Select
    w380 = 100  # Wait_Time
    # "Producer"
    n134 = event shown="[0] Timeout" {
      selector: _ -> [_ _ _ _ _ _ _ _ _ _]
      dyn-events: _ -> [_ _ _ _ _ _ _ _ _ _]
      timeout: w380 -> [_ _ _ _ _ _ _ _ _ _]
      tunnel: w381 -> [w393 w413 w423 w427 w435 w443 w448 w455 w459 w464]
      tunnel: [w382 w406 w420 w424 w429 w437 w445 w452 w456 w460] -> w377
      event Timeout {
        w390 = Queue_Operation_Select."Enqueue_N"  # Queue_Operation_Select
        w391 = Timer_Operation_Select."Time_Out?"  # Timer_Select
        # "Check for timer"
        n135 = event-data() -> ()  [unwired: 1 in, 1 out]
        n136 = call "Timer.vi"("Error_In"=w393, "Timer_Select"=w391) -> ("Time_Out?"=w388:bool, "Time"=w387:dbl, "Start?"=w384:bool, "Error_Out"=w392:errorcluster)  [unwired: 10 in]
        n137 = Build Array(w388, w384) -> (w385:bool[])
        n138 = Boolean Array To Number(Boolean array=w385) -> (number=w383:u32)
        n139 = case shown="2" w383 {
          tunnel: w392 -> [w394 w403 w405]
          tunnel: [w394 w403 w405] -> w389
          tunnel: [_ w400 w404] -> w386
          tunnel: w387 -> [_ w402 _]
          frame 0, Default {
          }
          frame 2 {
            w395 = T4 {"State"="", "Event_Data"=variant} ("State_and_Data_In")
            # "If the timer started, update FP and log"
            n140 = To Variant(anything=w402) -> (Variant=w398:variant)
            n141 = Bundle By Name(cluster=w395, "State"="FP_Update", "Event_Data"=w398) -> (w401:T4)
            n142 = Bundle By Name(cluster=w395, "State"="Log_the_Data", "Event_Data"=w398) -> (w396:T4)
            n143 = Build Array(w401, w396) -> (w400:T4[])
          }
          frame 3 {
            w404 = T4[] [{"State"="Time_Out?", "Event_Data"=variant}]  # States_and_Data
            # "If Timer timeout, jump to timeout"
          }
        }
        n144 = call "Queue_Driver.vi"("State_and_Data_In_N"=w386, "Error_In"=w389, "Queue_Operation_Select"=w390) -> ("Error_Out"=w382:errorcluster)  [unwired: 11 in, 1 out]
      }
      event "Run_Interlock", "Boiler_Reset": Value Change {
        # "Starts the Reset and lockout, if run interlocked"
        n145 = event-data() -> ()  [unwired: 1 in, 1 out]
        n146 = Build Array("Boiler_Reset", "Run_Interlock") -> (w411:bool[])
        n147 = Boolean Array To Number(Boolean array=w411) -> (number=w410:u32)
        n148 = case shown="3" w410 {
          tunnel: w413 -> [w415 w417 w419]
          tunnel: [w415 w417 w419] -> w412
          tunnel: [_ w416 w418] -> w408
          frame Default {
          }
          frame 0 {
            w416 = T4 {"State"="Shutdown_and_Purge", "Event_Data"=variant}  # State_and_Data_In
            # "Jump to Shutdown_and_Purge if run interlock opened"
          }
          frame 3 {
            w418 = T4 {"State"="Reset_Lockout", "Event_Data"=variant}  # State_and_Data_In
            # "Jump to Reset lockout, if run interlock closed"
          }
        }
        n149 = call "Queue_Driver.vi"("State_and_Data_In"=w408, "Error_In"=w412, "Queue_Operation_Select"=Queue_Operation_Select."Enqueue") -> ("Error_Out"=w406:errorcluster)  [unwired: 11 in, 1 out]
      }
      event "Start_Sequence": Value Change {
        w422 = Queue_Operation_Select."Enqueue"  # Queue_Operation_Select
        # "Starts the Pre Purge event"
        n150 = event-data() -> ()  [unwired: 1 in, 1 out]
        n151 = call "Queue_Driver.vi"("State_and_Data_In"=T4 {"State"="Pre_Purge", "Event_Data"=variant}, "Error_In"=w423, "Queue_Operation_Select"=w422) -> ("Error_Out"=w420:errorcluster)  [unwired: 11 in, 1 out]
      }
      event "Pilot": Value Change {
        w425 = T4 {"State"="Ignition", "Event_Data"=variant}  # State_and_Data_In
        w426 = Queue_Operation_Select."Enqueue"  # Queue_Operation_Select
        # "Starts the ignition event"
        n152 = event-data() -> ()  [unwired: 1 in, 1 out]
        n153 = call "Queue_Driver.vi"("State_and_Data_In"=w425, "Error_In"=w427, "Queue_Operation_Select"=w426) -> ("Error_Out"=w424:errorcluster)  [unwired: 11 in, 1 out]
      }
      event "Flame_Sensor_Value": Value Change {
        w432 = "Prove_the_Pilot"  # State
        w434 = Queue_Operation_Select."Enqueue"  # Queue_Operation_Select
        # "Starts Prove the Pilot event"
        n154 = event-data() -> ()  [unwired: 1 in, 1 out]
        n155 = To Variant(anything="Flame_Sensor_Value") -> (Variant=w430:variant)
        n156 = Bundle By Name(cluster=T4 {"State"="", "Event_Data"=variant} ("State_and_Data_In"), "State"=w432, "Event_Data"=w430) -> (w433:T4)
        n157 = call "Queue_Driver.vi"("State_and_Data_In"=w433, "Error_In"=w435, "Queue_Operation_Select"=w434) -> ("Error_Out"=w429:errorcluster)  [unwired: 11 in, 1 out]
      }
      event "Forced_Draft_Fan": Value Change {
        w442 = Queue_Operation_Select."Enqueue"  # Queue_Operation_Select
        # "Starts the Start and run event"
        n158 = event-data() -> ()  [unwired: 1 in, 1 out]
        n159 = To Variant(anything="Forced_Draft_Fan") -> (Variant=w438:variant)
        n160 = Bundle By Name(cluster=T4 {"State"="", "Event_Data"=variant} ("State_and_Data_In"), "State"="Start_and_Run", "Event_Data"=w438) -> (w441:T4)
        n161 = call "Queue_Driver.vi"("State_and_Data_In"=w441, "Error_In"=w443, "Queue_Operation_Select"=w442) -> ("Error_Out"=w437:errorcluster)  [unwired: 11 in, 1 out]
      }
      event "Fuel_Control_Valve": Value Change {
        w449 = "Start_and_Run_Cont"  # State
        w451 = Queue_Operation_Select."Enqueue"  # Queue_Operation_Select
        # "Starts the Start and run event Cont"
        n162 = event-data() -> ()  [unwired: 1 in, 1 out]
        n163 = To Variant(anything="Fuel_Control_Valve") -> (Variant=w446:variant)
        n164 = Bundle By Name(cluster=T4 {"State"="", "Event_Data"=variant} ("State_and_Data_In"), "State"=w449, "Event_Data"=w446) -> (w450:T4)
        n165 = call "Queue_Driver.vi"("State_and_Data_In"=w450, "Error_In"=w448, "Queue_Operation_Select"=w451) -> ("Error_Out"=w445:errorcluster)  [unwired: 11 in, 1 out]
      }
      event "Shutdown": Value Change {
        w453 = T4 {"State"="Shutdown_and_Purge", "Event_Data"=variant}  # State_and_Data_In
        w454 = Queue_Operation_Select."Enqueue"  # Queue_Operation_Select
        # "Shutdown the system"
        n166 = event-data() -> ()  [unwired: 1 in, 1 out]
        n167 = call "Queue_Driver.vi"("State_and_Data_In"=w453, "Error_In"=w455, "Queue_Operation_Select"=w454) -> ("Error_Out"=w452:errorcluster)  [unwired: 11 in, 1 out]
      }
      event "Stop": Value Change {
        w457 = T4 {"State"="Exit", "Event_Data"=variant}  # State_and_Data_In
        w458 = Queue_Operation_Select."Enqueue"  # Queue_Operation_Select
        # "If stop pressed, jump to Exit"
        n168 = event-data() -> ()  [unwired: 1 in, 1 out]
        n169 = call "Queue_Driver.vi"("State_and_Data_In"=w457, "Error_In"=w459, "Queue_Operation_Select"=w458) -> ("Error_Out"=w456:errorcluster)  [unwired: 11 in, 1 out]
      }
      event Panel Close? {
        w462 = T4 {"State"="Exit", "Event_Data"=variant}  # State_and_Data_In
        w463 = Queue_Operation_Select."Enqueue"  # Queue_Operation_Select
        # "If panel closed, Jump to Exit"
        n170 = event-data() -> ()  [unwired: 1 in, 1 out]
        n171 = call "Queue_Driver.vi"("State_and_Data_In"=w462, "Error_In"=w464, "Queue_Operation_Select"=w463) -> ("Error_Out"=w460:errorcluster)  [unwired: 11 in, 1 out]
        n172 = event-data ("Event Filter Node")("Discard?"=TRUE) -> ()  [unwired: 1 in, 1 out]
      }
    }
    n173 = call "Notifier_Driver.vi"("Error_In"=w377, "Notifier_Operation_Select"=w379) -> ("Latest_Notification"=w378:bool, "Error_Out"=w376:errorcluster)  [unwired: 12 in]
  }
  n174 = Merge Errors(w3, w4) -> (w2:errorcluster)
  n175 = call "Queue_Driver.vi"("Error_In"=w2, "Queue_Operation_Select"=w8) -> ("Error_Out"=w9:errorcluster)  [unwired: 12 in, 1 out]
  n176 = call "Queue_Driver.vi"("Error_In"=w9, "Queue_Operation_Select"=w6) -> ("Error_Out"=w7:errorcluster)  [unwired: 12 in, 1 out]
  n177 = call "Notifier_Driver.vi"("Error_In"=w7, "Notifier_Operation_Select"=w5) -> ("Error_Out"=→"Error_Out":errorcluster)  [unwired: 12 in, 1 out]
